vi "Download File.vi"(8 "error in (no error)":errorcluster, 9 "Connection Name":string, 10 "Local File Path":path, 11 "Remote File Path":string) -> (0 "error out":errorcluster, 3 "Return String":string)   [LabVIEW 2019, in "LabSFTP.lvlib"]
doc: "<License>This software is distributed under the BSD 3-Clause License. For the full license please see license.txt or visit www.labvolution.com/license</License>"
uses:
  LabSFTP.lvlib
  FGV State..enum.ctl
  C:/_Code/Development/Sub-Zero Functional Test/standard hardware/Universal Robots/UR LabVIEW Interface/LabSSH Library/References/LabSFTP.dll
  References/LabSFTP.dll
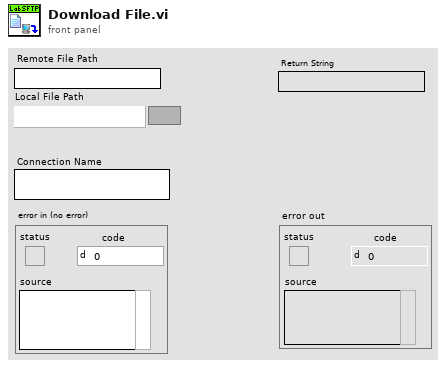
[diagram p1: front panel]
types:
  T1 = typedef "LabSFTP.lvlib/FGV State..enum.ctl" = enum16{"GET", "SET"}
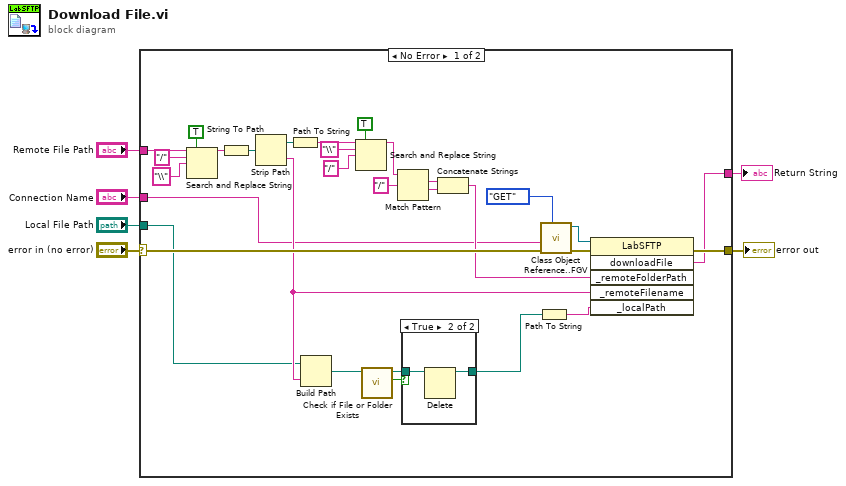
[diagram p0: block diagram]
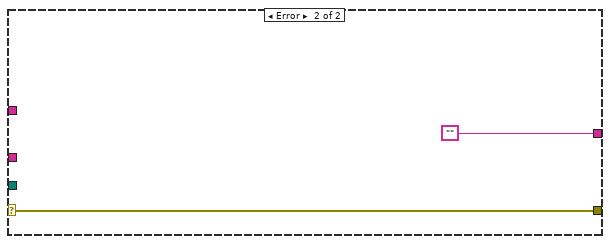
[diagram p3: hidden frame]
diagram:
  n1 = case shown="No Error" "error in (no error)" {
    selector: "error in (no error)" -> [w36 w41]
    tunnel: [w32 w41] -> w5
    tunnel: [w31 ""] -> w4
    tunnel: "Local File Path" -> [w9 _]
    tunnel: "Remote File Path" -> [w15 _]
    tunnel: "Connection Name" -> [w7 _]
    frame No Error {
      n2 = Search and Replace String(replace all?=TRUE ("replace all? (F)"), input string=w15, search string="/", replace string="\\" ("replace string (\"\")")) -> (result string=w19:string)  [unwired: 4 in, 3 out]
      n3 = String To Path(string=w19) -> (path=w20:path)
      n4 = Strip Path(path=w20) -> (stripped path=w21:path, name=w10:string)
      n5 = Path To String(path=w21) -> (string=w25:string)
      n6 = Build Path(base path=w9, name or relative path=w10) -> (appended path=w8:path)
      n7 = Search and Replace String(replace all?=TRUE ("replace all? (F)"), input string=w25, search string="\\", replace string="/" ("replace string (\"\")")) -> (result string=w27:string)  [unwired: 4 in, 3 out]
      n8 = call <vilib>:"Check if File or Folder Exists.vi"("path"=w8) -> ("file or folder exists?"=w13:bool, "dup path"=w12:path)  [unwired: 8 in, 1 out]
      n9 = Match Pattern(string=w27, regular expression="/") -> (match substring=w28:string, after substring=w29:string)  [unwired: 1 in, 2 out]
      n10 = case shown="True" w13 {
        tunnel: w12 -> [w37 w39]
        tunnel: [w37 w38] -> w11
        frame False {
        }
        frame True {
          n11 = Delete(path (use dialog)=w39) -> (deleted path=w38:path)  [unwired: 4 in, 2 out]
        }
      }
      n12 = Concatenate Strings(w28, w29) -> (w14:string)
      n13 = Path To String(path=w11) -> (string=w30:string)
      n14 = call "Class Object Reference..FGV.vi"("FGV State"=FGV_State..enum."GET", "error in (no error)"=w36, "Connection Name"=w7) -> ("error out"=w33:errorcluster, "LabSFTP ref out"=w34:refnum<k24>)  [unwired: 7 in]
      n15 = invoke class="LabSFTP" method="downloadFile"(reference=w34, error in=w33, "_remoteFolderPath"=w14, "_remoteFilename"=w10, "_localPath"=w30) -> (error out=w32:errorcluster, "downloadFile"=w31:string)  [unwired: 1 in, 4 out]
    }
    frame Error {
    }
  }
  "error out" <- w5
  "Return String" <- w4
